vi "Agilent ENA Series Application Limit Test.vi"() -> ()   [LabVIEW 2020]
doc: "Illustrates typical measuring task for a network analyzer and limit tests associated with the measurement. It measures a band-pass filter (center frequency: 947.5 MHz), and calculates and displays its bandwidth, insertion loss, and so on. \n\n<B>Note:</B>\n(1) For this function you must set DUT on instrument.\n(2) The limit tests must be loaded from a file."
uses:
  <instrlib>/Agilent ENA Series/Agilent ENA Series.lvlib
panel:
  in  "Save State (F: Disable)":bool
  out "Limit Fail":bool
  in  "Channel (1)":i32=1
  in  "File Name ()":string
  in  "Reset? (T: Yes)":bool=TRUE
  in  "ID Query? (T: Yes)":bool=TRUE
  out "High":dbl
  out "Low":dbl
  out "Center Frequency":dbl format="%^.2e"
  out "Q Value":dbl format="%^.2e"
  out "Loss":dbl format="%^.2e"
  out "Bandwidth":dbl format="%^.2e"
  in  "VISA resource name":refnum<visa-resource-name>
  # "(c) 2005-2021 National Instruments.  ALL RIGHTS RESERVED."
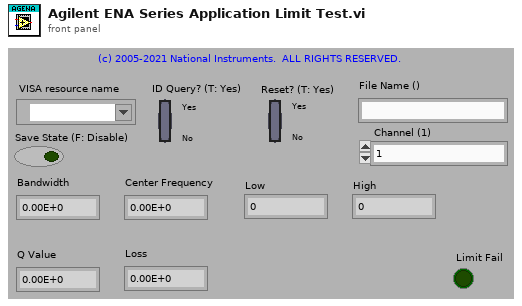
[diagram p1: front panel]
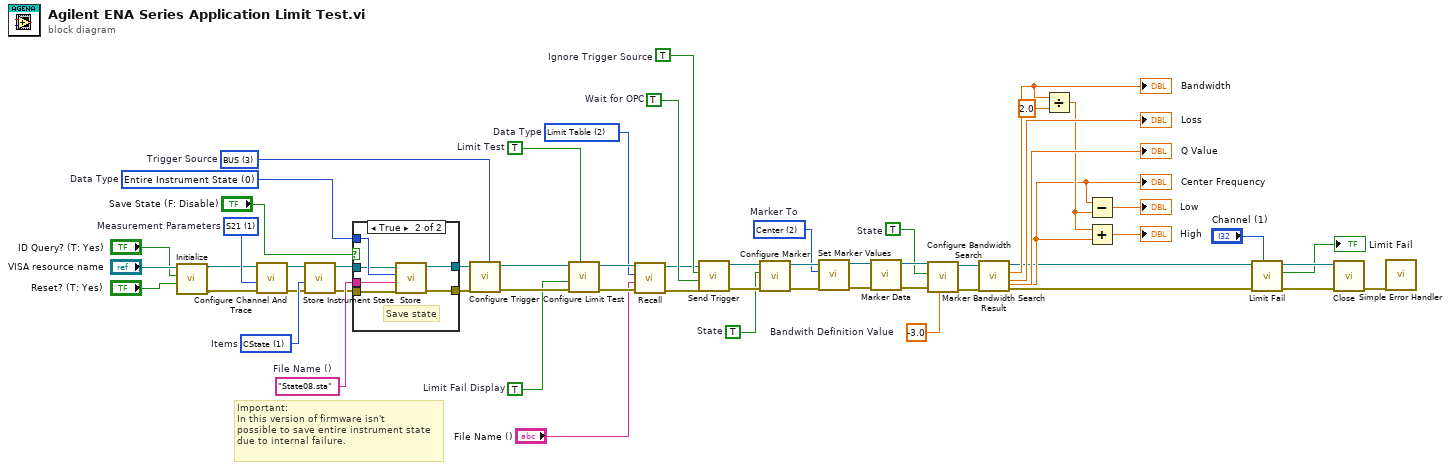
[diagram p0: block diagram]
diagram:
  w6 = u16 1 items=["S11", "S21", "S31", "S41", "S12", "S22", "S32", "S42", "S13", "S23", "S33", "S43", "S14", "S24", "S34", "S44", "A", "B", "C", "D", "R1", "R2", "R3", "R4"]  # Measurement Parameters
  w20 = u16 2 items=["Entire Instrument State", "Segment Sweep Table", "Limit Table", "Power Sensor A", "Power Sensor B", "VBA Project", "Loss Compensation Table 1", "Loss Compensation Table 2", "Loss Compensation Table 3", "Loss Compensation Table 4"]  # Data Type
  w23 = TRUE  # Limit Fail Display
  w7 = TRUE  # Limit Test
  w44 = -3.0  # Bandwith Definition Value
  w45 = TRUE  # State
  w50 = u16 2 items=["Start", "Stop", "Center", "Reference", "Electrical Delay"]  # Marker To
  w53 = TRUE  # State
  w56 = TRUE  # Wait for OPC
  w57 = TRUE  # Ignore Trigger Source
  w58 = u16 3 items=["Internal", "External", "Manual", "BUS"]  # Trigger Source
  w30 = "State08.sta"  # File Name ()
  w31 = u16 0 items=["Entire Instrument State", "Formatted Data Array", "Image On The LCD Display", "Segment Sweep Table", "Limit Table", "Power Sensor A", "Power Sensor B", "VBA Project", "Loss Compensation Table 1", "Loss Compensation Table 2", "Loss Compensation Table 3", "Loss Compensation Table 4"]  # Data Type
  w10 = u16 1 items=["State", "CState", "Dstate", "CDState"]  # Items
  # "Important:\nIn this version of firmware isn't \npossible to save entire instrument state\ndue to internal failure."
  n1 = call <instrlib>:"Initialize.vi"("Reset? (T: Yes)"="Reset? (T: Yes)", "ID Query? (T: Yes)"="ID Query? (T: Yes)", "VISA resource name"="VISA resource name") -> ("error out"=w4:errorcluster, "VISA resource name out"=w5:refnum<visa-resource-name>)  [unwired: 7 in]
  n2 = call <instrlib>:"Configure Channel And Trace.vi"("error in (no error)"=w4, "Measurement Parameters (0: S11)"=w6, "VISA resource name"=w5) -> ("error out"=w2:errorcluster, "VISA resource name out"=w3:refnum<visa-resource-name>)  [unwired: 7 in]
  n3 = call <instrlib>:"Store Instrument State.vi"("error in (no error)"=w2, "Items (3: CDState)"=w10, "VISA resource name"=w3) -> ("error out"=w8:errorcluster, "VISA resource name out"=w9:refnum<visa-resource-name>)  [unwired: 7 in]
  n4 = case shown="True" "Save State (F: Disable)" {
    tunnel: w31 -> [_ w66]
    tunnel: w30 -> [_ w65]
    tunnel: w9 -> [w60 w64]
    tunnel: [w60 w63] -> w29
    tunnel: w8 -> [w59 w62]
    tunnel: [w59 w61] -> w28
    frame False {
      # "Don't save"
    }
    frame True {
      # "Save state"
      n5 = call <instrlib>:"Store.vi"("error in (no error)"=w62, "File Name ()"=w65, "Data Type (0: Entire Instrument State)"=w66, "VISA resource name"=w64) -> ("error out"=w61:errorcluster, "VISA resource name out"=w63:refnum<visa-resource-name>)  [unwired: 6 in]
    }
  }
  n6 = call <instrlib>:"Configure Trigger.vi"("Trigger Source (0: Internal)"=w58, "error in (no error)"=w28, "VISA resource name"=w29) -> ("error out"=w25:errorcluster, "VISA resource name out"=w24:refnum<visa-resource-name>)  [unwired: 7 in]
  n7 = call <instrlib>:"Configure Limit Test.vi"("Limit Test (F: Disable)"=w7, "error in (no error)"=w25, "Limit Fail Display (F: Disable)"=w23, "VISA resource name"=w24) -> ("error out"=w22:errorcluster, "VISA resource name out"=w21:refnum<visa-resource-name>)  [unwired: 6 in]
  n8 = call <instrlib>:"Recall.vi"("error in (no error)"=w22, "File Name ()"="File Name ()", "Data Type (0: Entire Instrument State)"=w20, "VISA resource name"=w21) -> ("error out"=w18:errorcluster, "VISA resource name out"=w17:refnum<visa-resource-name>)  [unwired: 6 in]
  n9 = call <instrlib>:"Send Trigger.vi"("error in (no error)"=w18, "Wait for OPC (F: Do not Wait)"=w56, "Ignore Trigger Source (F: Do not Ignore)"=w57, "VISA resource name"=w17) -> ("error out"=w54:errorcluster, "VISA resource name out"=w55:refnum<visa-resource-name>)  [unwired: 6 in]
  n10 = call <instrlib>:"Configure Marker.vi"("error in (no error)"=w54, "Marker State (F: Disabled)"=w53, "VISA resource name"=w55) -> ("error out"=w51:errorcluster, "VISA resource name out"=w52:refnum<visa-resource-name>)  [unwired: 7 in]
  n11 = call <instrlib>:"Set Marker Values.vi"("error in (no error)"=w51, "Marker To (0: Start)"=w50, "VISA resource name"=w52) -> ("error out"=w48:errorcluster, "VISA resource name out"=w49:refnum<visa-resource-name>)  [unwired: 7 in]
  n12 = call <instrlib>:"Marker Data.vi"("error in (no error)"=w48, "VISA resource name"=w49) -> ("error out"=w46:errorcluster, "VISA resource name out"=w47:refnum<visa-resource-name>)  [unwired: 5 in, 3 out]
  n13 = call <instrlib>:"Configure Bandwidth Search.vi"("Bandwidth Definition Value (-3.0)"=w44, "error in (no error)"=w46, "Result Display State (F: Disable)"=w45, "VISA resource name"=w47) -> ("error out"=w42:errorcluster, "VISA resource name out"=w43:refnum<visa-resource-name>)  [unwired: 6 in]
  n14 = call <instrlib>:"Marker Bandwidth Search Result.vi"("error in (no error)"=w42, "VISA resource name"=w43) -> ("error out"=w16:errorcluster, "Loss"=→"Loss":dbl, "Bandwidth"=w39:dbl, "VISA resource name out"=w15:refnum<visa-resource-name>, "Q Value"=→"Q Value":dbl, "Center Frequency"=w35:dbl)  [unwired: 4 in]
  "Bandwidth" <- w39
  "Center Frequency" <- w35
  n15 = Divide(x=w39, y=2.0) -> (x/y=w36:dbl)
  n16 = Subtract(x=w35, y=w36) -> (x-y=→"Low":dbl)
  n17 = Add(x=w36, y=w35) -> (x+y=→"High":dbl)
  n18 = call <instrlib>:"Limit Fail.vi"("Channel (1)"="Channel (1)", "error in (no error)"=w16, "VISA resource name"=w15) -> ("error out"=w14:errorcluster, "Limit Fail"=→"Limit Fail":bool, "VISA resource name out"=w13:refnum<visa-resource-name>)  [unwired: 6 in]
  n19 = call <instrlib>:"Close.vi"("error in (no error)"=w14, "VISA resource name"=w13) -> ("error out"=w33:errorcluster)  [unwired: 9 in]
  n20 = call <vilib>:"Simple Error Handler.vi"("error in (no error)"=w33) -> ()  [unwired: 4 in, 5 out]
